vi "increment folder name.vi"(11 "Image folder":path) -> (3 "appended path":path)   [LabVIEW 2015, in "Camera SubVIs.lvlib"]
uses:
  Camera SubVIs.lvlib
panel:
  out "concatenated string":string
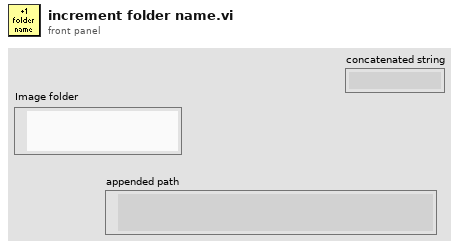
[diagram p1: front panel]
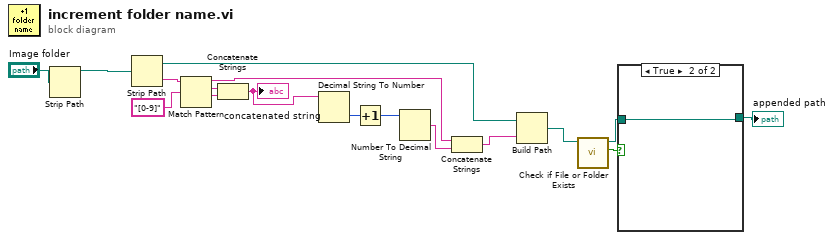
[diagram p0: block diagram]
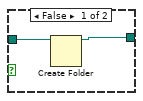
[diagram p2: hidden frame]
diagram:
  n1 = Strip Path(path="Image folder") -> (stripped path=w5:path)  [unwired: 1 out]
  n2 = Strip Path(path=w5) -> (stripped path=w7:path, name=w17:string)
  n3 = Match Pattern(string=w17, regular expression="[0-9]") -> (before substring=w10:string, match substring=w15:string, after substring=w14:string)  [unwired: 1 in, 1 out]
  n4 = Concatenate Strings(w15, w14) -> (w13:string)
  "concatenated string" <- w13
  n5 = Decimal String To Number(string=w13) -> (number=w12:i32)  [unwired: 2 in, 1 out]
  n6 = Increment(x=w12) -> (x+1=w11:i32)
  n7 = Number To Decimal String(number=w11) -> (decimal integer string=w9:string)  [unwired: 1 in]
  n8 = Concatenate Strings(w10, w9) -> (w8:string)
  n9 = Build Path(base path=w7, name or relative path=w8) -> (appended path=w4:path)
  n10 = call <vilib>:"Check if File or Folder Exists.vi"("path"=w4) -> ("file or folder exists?"=w3:bool, "dup path"=w2:path)  [unwired: 8 in, 1 out]
  n11 = case shown="True" w3 {
    tunnel: w2 -> [w19 w20]
    tunnel: [w18 w20] -> w1
    frame False {
      n12 = Create Folder(path (use dialog)=w19) -> (created path=w18:path)  [unwired: 2 in, 2 out]
    }
    frame True {
    }
  }
  "appended path" <- w1
